vi "Initialize Attributes Core.vi"(8 "error in (no error)":errorcluster, 10 "Attribute Data":variant, 11 "BNT_XtGraph in":refnum<class "BNT_XtGraph.lvclass">) -> (0 "error out":errorcluster, 2 "MandatoryParameters":cluster{"Parameter":string, "found?":bool}[](array[cluster]), 3 "BNT_XtGraph out":refnum<class "BNT_XtGraph.lvclass">)   [LabVIEW 2019, in "BNT_XtGraph.lvlib" / "BNT_XtGraph.lvclass"]
doc: "Initialize object attribute.\n\nUnique resources should be allocated elsewhere!"
uses:
  BNT_XtGraph.lvclass
  CSPP_Core/Libraries/Utilities/CSPP_Utilities.lvlib
  CSPP_Core/Actors/CSPP_BaseActor/CSPP_BaseActor.lvclass
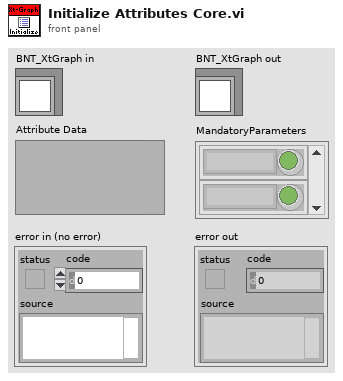
[diagram p1: front panel]
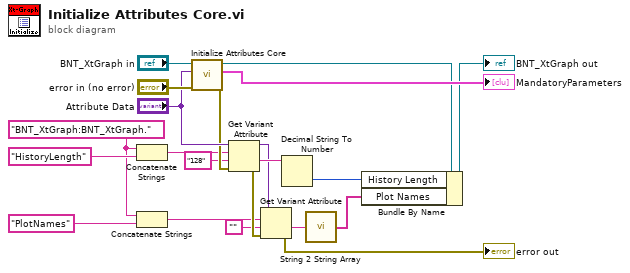
[diagram p0: block diagram]
diagram:
  w8 = "BNT_XtGraph:BNT_XtGraph."
  n1 = Concatenate Strings(w8, "HistoryLength") -> (w15:string)
  n2 = Concatenate Strings(w8, "PlotNames") -> (w4:string)
  n3 = call-parent "Initialize Attributes Core.vi"("error in (no error)"="error in (no error)", "Attribute Data"="Attribute Data", "CSPP_BaseActor in"="BNT_XtGraph in") -> ("error out"=w17:errorcluster, "MandatoryParameters"=→"MandatoryParameters":cluster{"Parameter":string, "found?":bool}[], "CSPP_BaseActor out"=w13:refnum<class "BNT_XtGraph.lvclass">)  [unwired: 6 in]
  n4 = Get Variant Attribute(Variant="Attribute Data", name=w15, default value (empty Variant)="128", error in=w17) -> (duplicate Variant=w7:variant, value=w11:string, error out=w6:errorcluster)  [unwired: 1 out]
  n5 = Get Variant Attribute(Variant=w7, name=w4, default value (empty Variant)="", error in=w6) -> (value=w2:string, error out=→"error out":errorcluster)  [unwired: 2 out]
  n6 = Decimal String To Number(string=w11) -> (number=w10:i32)  [unwired: 2 in, 1 out]
  n7 = call "String 2 String Array.vi"("String"=w2) -> ("Substrings"=w1:string[])  [unwired: 1 in]
  n8 = Bundle By Name(cluster=w13, "History Length"=w10, "Plot Names"=w1) -> (→"BNT_XtGraph out":refnum<class "BNT_XtGraph.lvclass">)
